vi "close.vi"(8 "error in (no error)":errorcluster, 11 "ScriptEditorV2 in":refnum<class "ScriptEditorV2.lvclass">) -> (0 "error out":errorcluster, 2 "close":bool, 3 "ScriptEditorV2 out":refnum<class "ScriptEditorV2.lvclass">)   [LabVIEW 2011, in "Views.lvlib" / "ScriptEditor.lvlib" / "ScriptEditorV2.lvclass"]
uses:
  ScriptEditorV2.lvclass
  ScriptEditorV2.lvclass/ScriptEditorV2.ctl
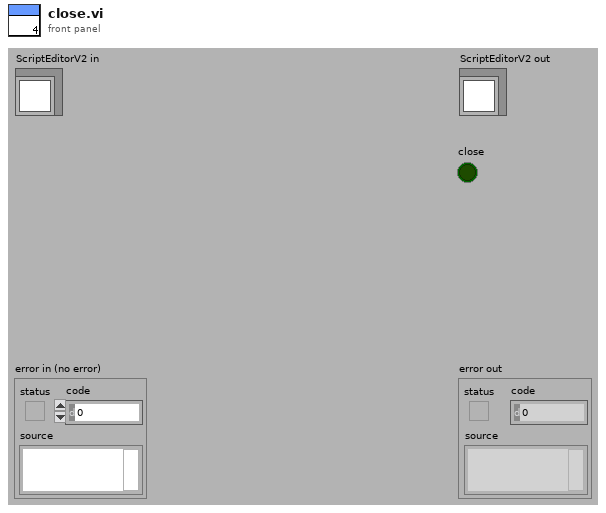
[diagram p1: front panel]
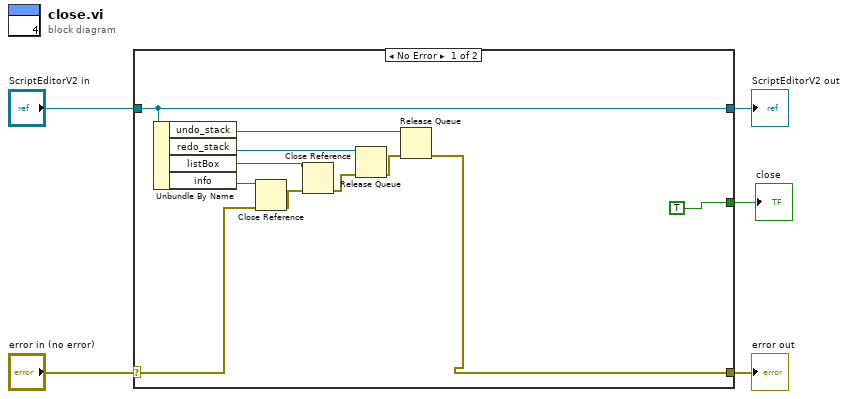
[diagram p0: block diagram]
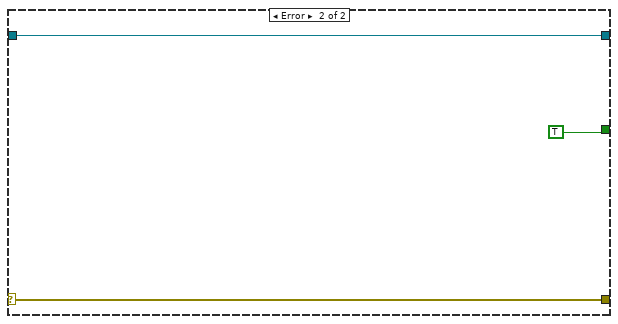
[diagram p2: hidden frame]
diagram:
  n1 = case shown="No Error" "error in (no error)" {
    selector: "error in (no error)" -> [w7 w19]
    tunnel: [w6 w19] -> w4
    tunnel: [w15 w18] -> w2
    tunnel: "ScriptEditorV2 in" -> [w15 w18]
    tunnel: [TRUE TRUE] -> w1
    frame No Error {
      n2 = Unbundle By Name(w15) -> ("undo_stack"=w9:refnum<queue>, "redo_stack"=w10:refnum<queue>, "listBox"=w13:refnum<vi>, "info"=w14:refnum<vi>)
      n3 = Close Reference(reference=w14, error in (no error)=w7) -> (error out=w12:errorcluster)
      n4 = Close Reference(reference=w13, error in (no error)=w12) -> (error out=w11:errorcluster)
      n5 = Release Queue(queue=w10, error in (no error)=w11) -> (error out=w8:errorcluster)  [unwired: 1 in, 2 out]
      n6 = Release Queue(queue=w9, error in (no error)=w8) -> (error out=w6:errorcluster)  [unwired: 1 in, 2 out]
    }
    frame Error {
    }
  }
  "error out" <- w4
  "ScriptEditorV2 out" <- w2
  "close" <- w1
